vi "_Construct.vi"(8 "error in (no error)":errorcluster, 11 "ChanSel init":string) -> (0 "error out":errorcluster, 3 "SingleIndi out":refnum<class "SingleIndi.lvclass">)   [LabVIEW 2020, in "SingleIndi.lvlib" / "SingleIndi.lvclass"]
uses:
  SingleIndi.lvclass
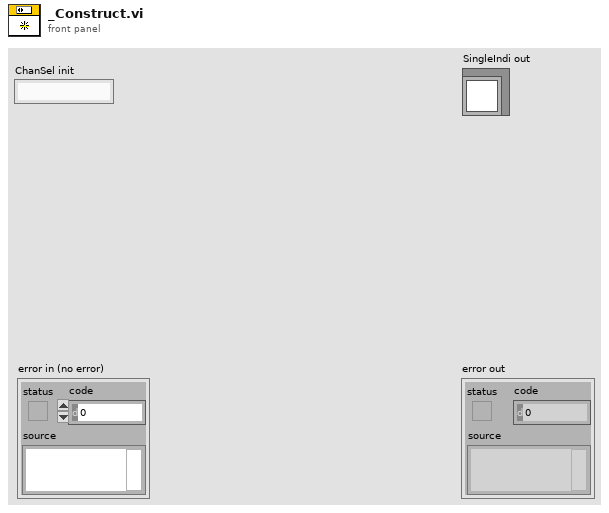
[diagram p1: front panel]
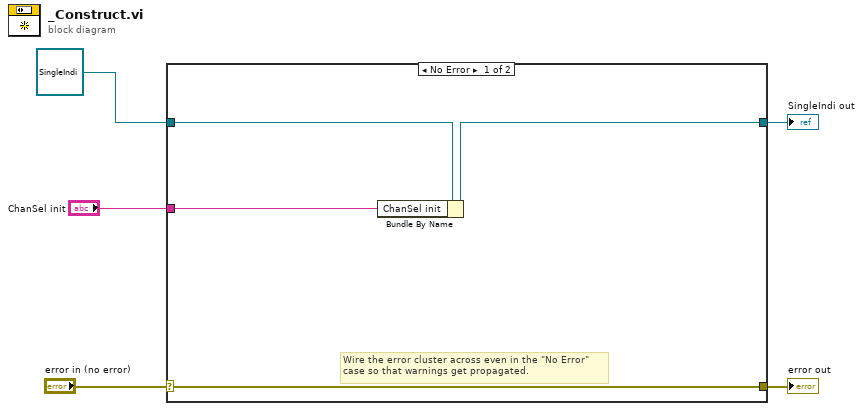
[diagram p0: block diagram]
diagram:
  n1 = case shown="No Error" "error in (no error)" {
    selector: "error in (no error)" -> [w8 w11]
    tunnel: [w8 w11] -> w4
    tunnel: [w7 w10] -> w2
    tunnel: refnum<class "SingleIndi.lvclass"> refnum ("SingleIndi in") -> [w9 w10]
    tunnel: "ChanSel init" -> [w6 _]
    frame No Error {
      # "Wire the error cluster across even in the \"No Error\"\ncase so that warnings get propagated."
      n2 = Bundle By Name(cluster=w9, "ChanSel init"=w6) -> (w7:refnum<class "SingleIndi.lvclass">)
    }
    frame Error {
    }
  }
  "error out" <- w4
  "SingleIndi out" <- w2
